vi "SubModule Read Data.vi"(8 "error in (no error)":errorcluster, 11 "Nikon in":refnum<class "Nikon.lvclass">) -> (0 "error out":errorcluster, 1 "Data":string[](array[string]), 3 "Nikon out":refnum<class "Nikon.lvclass">)   [LabVIEW 2021, in "Nikon.lvclass"]
uses:
  Nikon.lvclass
  C:/Projects/InstrPanel/Classes/Camera/Camera.lvclass
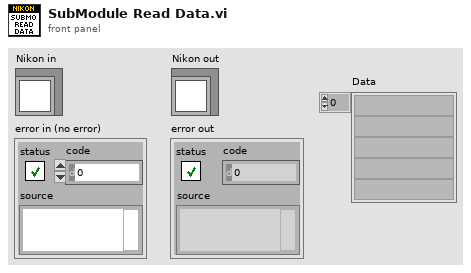
[diagram p1: front panel]
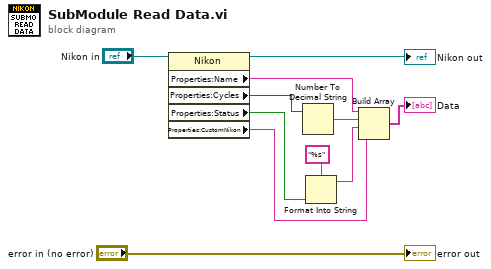
[diagram p0: block diagram]
diagram:
  n1 = property class="Nikon"(reference="Nikon in") -> (reference out=→"Nikon out":refnum<class "Nikon.lvclass">, "Properties:Name"=w4:string, "Properties:Cycles"=w3:i32, "Properties:Status"=w1:bool, "Properties:CustomNikon"=w2:string)  [unwired: 1 in, 1 out]
  n2 = Number To Decimal String(number=w3) -> (decimal integer string=w9:string)  [unwired: 1 in]
  n3 = Format Into String(format string="%s", w1) -> (resulting string=w8:string)  [unwired: 2 in, 1 out]
  n4 = Build Array(w4, w9, w8, w2) -> (→"Data":string[])
  "error out" <- "error in (no error)"
